vi "test_Read FXP Register Value.vi"(8 "error in (no error)":errorcluster, 11 "TestCase in":refnum<class "FPGA Register IO Tests.lvclass">=refnum) -> (0 "error out":errorcluster, 3 "TestCase out":refnum<class "FPGA Register IO Tests.lvclass">)   [LabVIEW 2026, in "FPGA Register IO Tests.lvclass"]
uses:
  FPGA Register IO Tests.lvclass
  FPGA Register IO Tests.lvclass/FPGA Register IO Tests.ctl
  APIs/FPGA Register IO/FPGA Register IO.lvlib
  <vilib>/rvi/interface/nirviCloseFPGA/nirviCloseFPGA.xnode
  <vilib>/FPGAPlugInAG/Dynamic/niLvFpga_Close_Dynamic.vi
  <vilib>/fxp/LVFixedPointRepRangeTypeDef.ctl
  <vilib>/fxp/LVFixedPointRepBitsTypeDef.ctl
  APIs/FPGA Register IO/TypeDefs/FXP Configuration.ctl
  APIs/FPGA Register IO/Read Methods/Read Data Register/Instances/Read FXP.vi
  Addon/Addon Engine/FPGA Addon Engine.lvlib
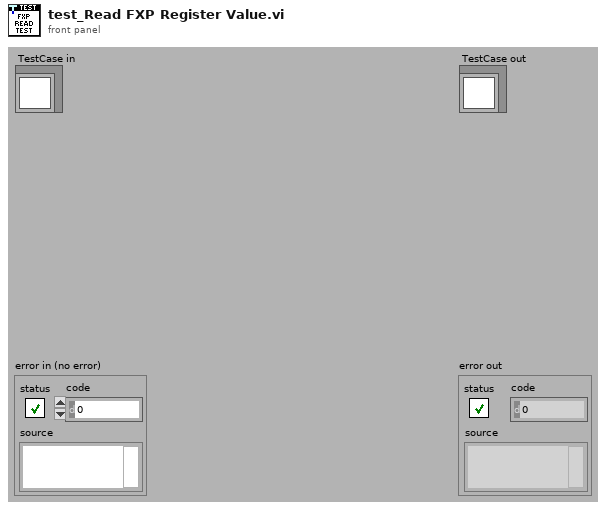
[diagram p1: front panel]
types:
  T1 = typedef "FPGA Register IO.lvlib/FXP Configuration.ctl" = cluster{"FXP Representation":T2, "FXP Range":T3}
  T2 = typedef "LVFixedPointRepBitsTypeDef.ctl" = cluster{"Signed":bool, "Word Length":u32, "Integer Word Length":i32}
  T3 = typedef "LVFixedPointRepRangeTypeDef.ctl" = cluster{"Range Min":dbl, "Range Max":dbl, "Delta":dbl}
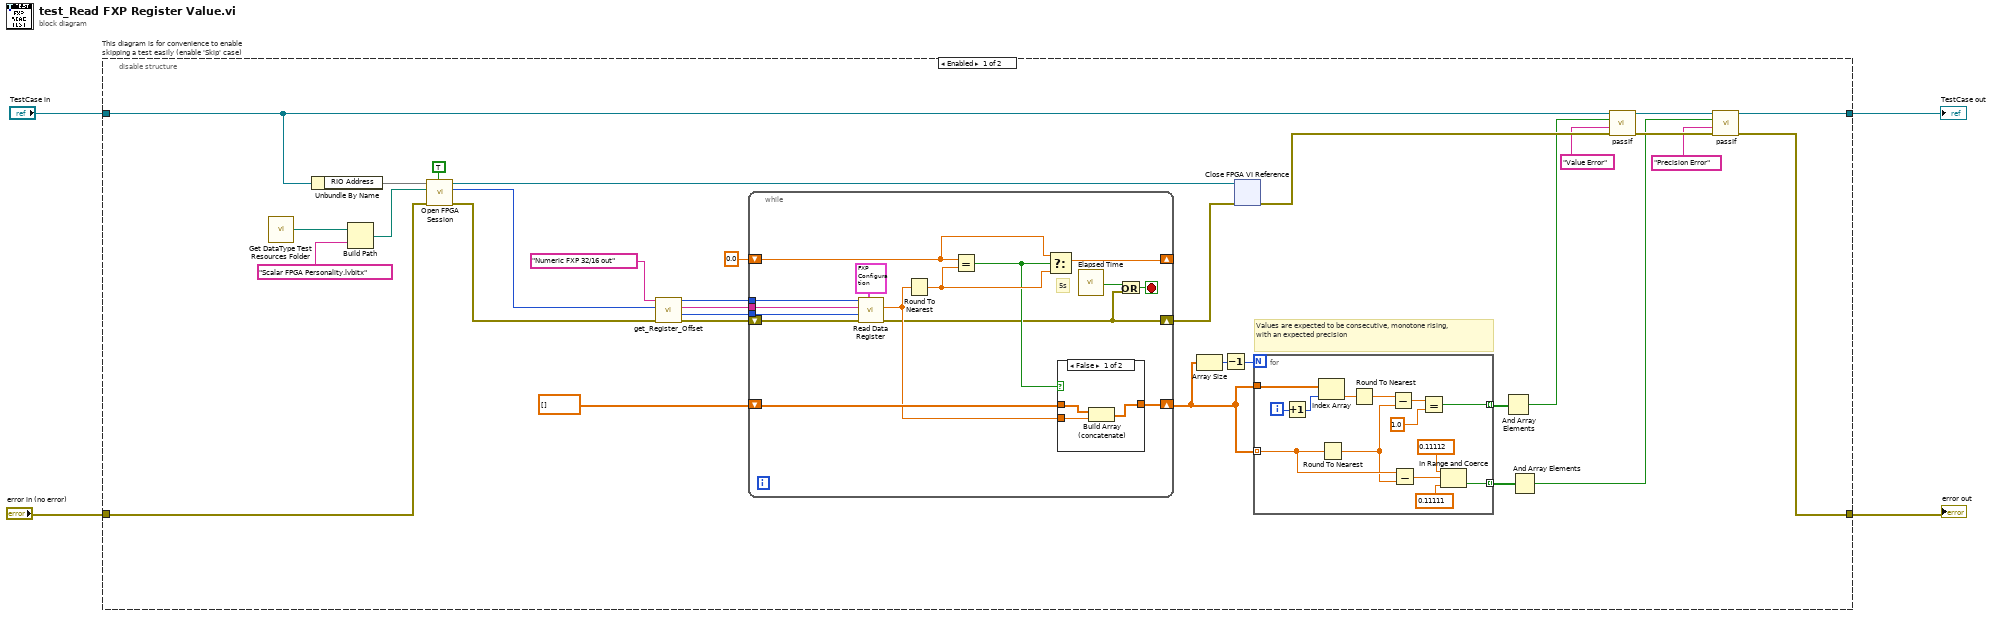
[diagram p0: block diagram]
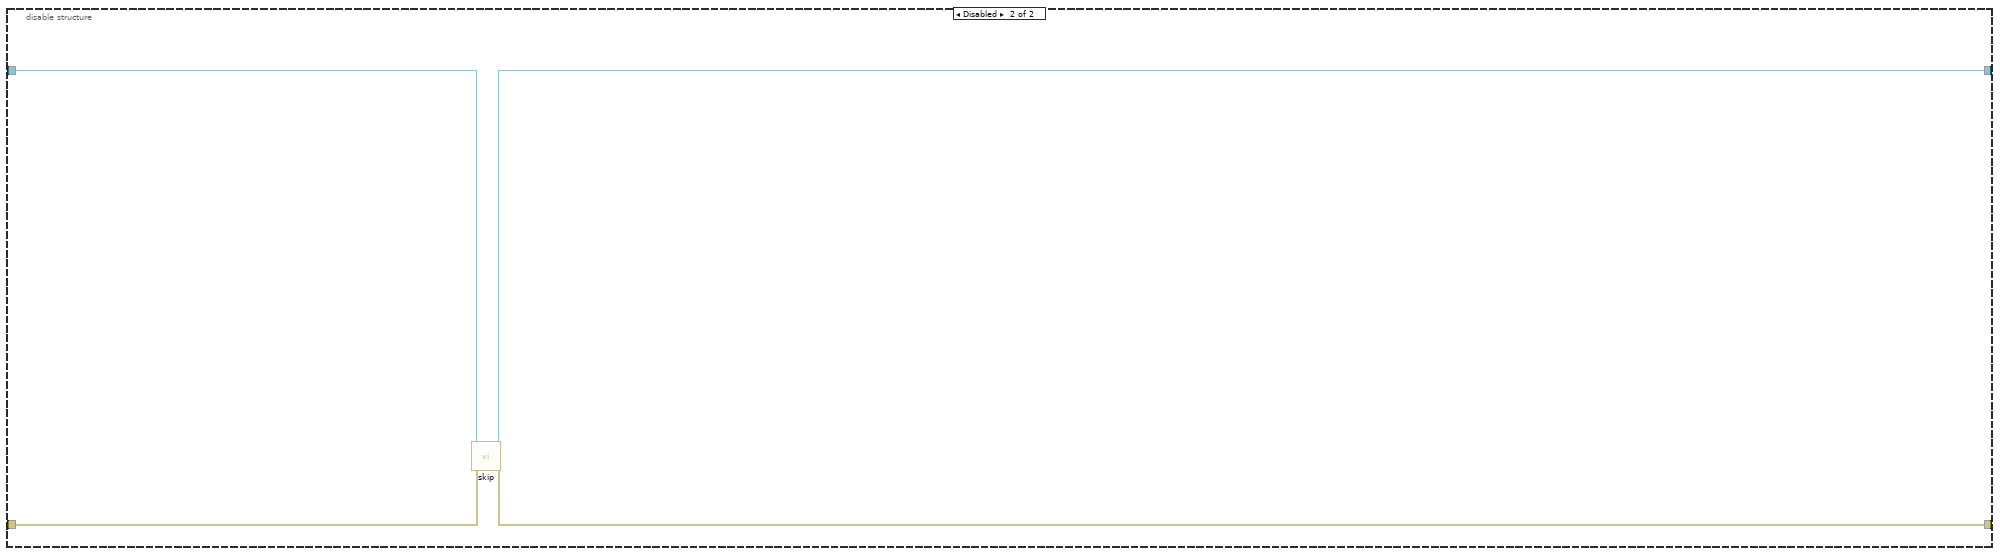
[diagram p3: hidden frame]
diagram:
  n1 = disable-structure "This diagram is for convenience to enable skipping a test easily (enable 'Skip' case)" shown="Enabled" {
    disable-tunnel: "TestCase in" -> [w22 w73]
    disable-tunnel: [w12 w71] -> w1
    disable-tunnel: [w13 w72] -> w3
    disable-tunnel: "error in (no error)" -> [w23 w70]
    frame Enabled {
      # "Values are expected to be consecutive, monotone rising, with an expected precision"
      n2 = call "Get DataType Test Resources Folder.vi"() -> ("path"=w20:path)
      n3 = Unbundle By Name(w22) -> ("RIO Address"=w25)
      n4 = Build Path(base path=w20, name or relative path="Scalar FPGA Personality.lvbitx") -> (appended path=w24:path)
      n5 = call "Open FPGA Session.vi"("run when loaded (T)"=TRUE ("Run When Loaded (T)"), "error in"=w23, "bitfile path"=w24, "device address"=w25) -> ("error out"=w30:errorcluster, "session out"=w9:u32, "bitfile reference out"=w29:refnum<k20>)  [unwired: 5 in]
      n6 = call "get_Register_Offset.vi"("error in (no error)"=w30, "session"=w9, "Name"="Numeric FXP 32/16 out" ("registerName")) -> ("error out"=w10:errorcluster, "RegisterOffset"=w5:u32, "Register Name"=w6:string, "session out"=w8:u32)  [unwired: 5 in]
      n7 = while {
        tunnel: w8 -> [w45]
        shift-right: [w39] -> w28
        shift-left: w10 -> [w44]
        shift-right: [w49] -> _
        shift-left: 0.0 ("DBL Value") -> [w51]
        shift-right: [w47] -> w31
        shift-left: dbl[] [] -> [w46]
        tunnel: w6 -> [w38]
        tunnel: w5 -> [w37]
        stop <- w41 stop-if-true
        # "5s"
        n8 = call-poly "Read Data Register.vi"("FXP Configuration"=T1 {"FXP Representation"={"Signed"=TRUE, "Word Length"=32, "Integer Word Length"=16}, "FXP Range"={"Range Min"=0.0, "Range Max"=0.0, "Delta"=1.52588e-05}}, "error in"=w44, "RegisterOffset"=w37, "register name"=w38, "session in"=w45) -> ("error out"=w39:errorcluster, "DBL Value"=w43:dbl)  [unwired: 4 in, 1 out]
        n9 = Round To Nearest(number=w43) -> (nearest integer value=w50:dbl)
        n10 = Equal?(x=w51, y=w50) -> (x = y?=w48:bool)
        n11 = Select(t=w51, s=w48, f=w50) -> (s? t:f=w49:dbl)
        n12 = case shown="False" w48 {
          tunnel: w43 -> [w54 _]
          tunnel: [w53 w55] -> w47
          tunnel: w46 -> [w52 w55]
          frame False {
            n13 = Build Array (concatenate)(w52, w54) -> (w53:dbl[])
          }
          frame True {
          }
        }
        n14 = call "Elapsed Time"() -> ("Time has Elapsed"=w40:bool)  [unwired: 12 in, 7 out]
        n15 = Or(x=w40, y=w39) -> (x .or. y?=w41:bool)
      }
      n16 = Array Size(array=w31) -> (size(s)=w32:i32)
      n17 = Decrement(x=w32) -> (x-1=w33:i32)
      n18 = xnode "Close FPGA VI Reference"("FPGA VI Reference In"=w29, "error in"=w28) -> ("error out"=w21:errorcluster)
      n19 = for {
        N: w33 -> [_]
        tunnel: w31 -> [w64] mode=indexing
        tunnel: w31 -> [w69]
        tunnel: [w60] -> w34 mode=indexing
        tunnel: [w57] -> w35 mode=indexing
        i -> [w68]
        n20 = Increment(x=w68) -> (x+1=w67:i32)
        n21 = Index Array(array=w69, index=w67) -> (element=w66:dbl)
        n22 = Round To Nearest(number=w64) -> (nearest integer value=w63:dbl)
        n23 = Round To Nearest(number=w66) -> (nearest integer value=w65:dbl)
        n24 = Subtract(x=w65, y=w63) -> (x-y=w62:dbl)
        n25 = Subtract(x=w64, y=w63) -> (x-y=w56:dbl)
        n26 = Equal?(x=w62, y=1.0) -> (x = y?=w60:bool)
        n27 = In Range and Coerce(upper limit=0.11112, x=w56, lower limit=0.11111 ("upper limit")) -> (In Range?=w57:bool)  [unwired: 1 out]
      }
      n28 = And Array Elements(Boolean array=w34) -> (logical AND=w19:bool)
      n29 = And Array Elements(Boolean array=w35) -> (logical AND=w15:bool)
      n30 = call-dynamic "passIf.vi"("error in (no error)"=w21, "message (\"\")"="Value Error" ("message (\"\")"), "pass"=w19, "TestCase in"=w22) -> ("error out"=w17:errorcluster, "TestCase out"=w16:refnum<class "FPGA Register IO Tests.lvclass">)  [unwired: 6 in]
      n31 = call-dynamic "passIf.vi"("error in (no error)"=w17, "message (\"\")"="Precision Error" ("message (\"\")"), "pass"=w15, "TestCase in"=w16) -> ("error out"=w13:errorcluster, "TestCase out"=w12:refnum<class "FPGA Register IO Tests.lvclass">)  [unwired: 6 in]
    }
    frame Disabled {
      # "skip test result while test is under development"
      n32 = call <vilib>:"skip.vi"("error in (no error)"=w70, "TestCase in"=w73) -> ("error out"=w72:errorcluster, "TestCase out"=w71:refnum<class "FPGA Register IO Tests.lvclass">)  [unwired: 8 in]
    }
  }
  "error out" <- w3
  "TestCase out" <- w1
